vi "Register with Manager.vi"(8 "error in (no error)":errorcluster, 11 "CIFCorePlugin in":refnum<class "CIFCorePlugin.lvclass">) -> (0 "error out":errorcluster, 3 "CIFCorePlugin out":refnum<class "CIFCorePlugin.lvclass">)   [LabVIEW 2021, in "CIFCorePlugin.lvclass"]
uses:
  CIFCorePlugin.lvclass
  CIFPluginManager/CIFPluginManager/gRPC/CIF_Manager_client/RPC Messages/cif_manager_RegisterData.ctl
  CIFPluginManager/CIFPluginManager/gRPC/CIF_Manager_client/RPC Messages/cif_common_ShortVersion.ctl
  CIFCorePlugin.lvclass/CIFCorePlugin.ctl
  Common/Typedef/Errors.ctl
  <vilib>/gRPC/LabVIEW gRPC Library/Shared/grpcId.ctl
  <vilib>/CIF Foundation/CIF Utilities/Errors/Append Error Location.vi
  CIFPluginManager/CIFPluginManager/gRPC/CIF_Manager_Client_Wrapper/CIFManagerClientWrapper.lvlib
  CIFUtilities/CIFConfigurationFile/CIF Configuration File.lvlib
  CIFPluginManager/CIFPluginManager/gRPC/CIF_Manager_client/CIF_Manager_client.lvlib
  Common/CIFCoreCommon.lvlib
  <vilib>/gRPC/LabVIEW gRPC Library/grpc-lvsupport-release.lvlib
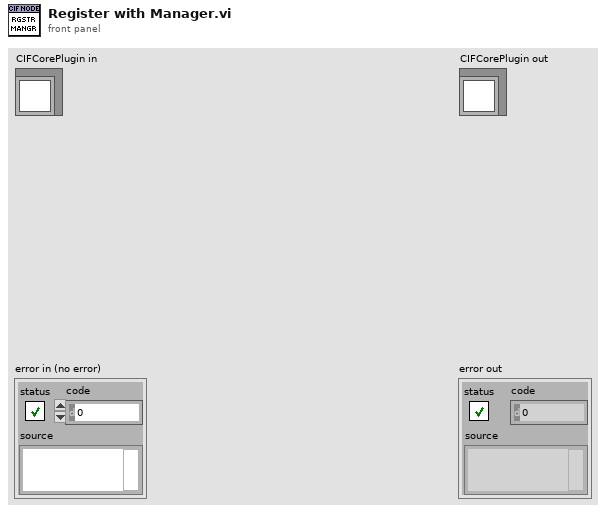
[diagram p1: front panel]
types:
  T1 = typedef "CIF_Manager_client.lvlib/cif_manager_RegisterData.ctl" = cluster{"plugin_name":string, "grpc_port":i32, "plugin_version":T2}
  T2 = typedef "CIF_Manager_client.lvlib/cif_common_ShortVersion.ctl" = cluster{"major":u32, "minor":u32, "fix":u32}
  T3 = typedef "grpc-lvsupport-release.lvlib/grpcId.ctl" = u64
  T4 = typedef "CIFCoreCommon.lvlib/Errors.ctl" = enum16{"Invalid Clock ID", "Long Sleep", "gRPC Server Not Found", "Config Parse", "Timestamp Wrap", "Delayed Execution", "Duplicate Channel", "Missing Channel", "Incorrect Type", "Flatten Error", "Unflatten Data", "Unique Name", "Plugin Not Found", "Plugin Type Not Found", "Plugin Version Not Found", "Manager Not Found", "Numerical Issue", "Time Jump", "Clock ID Match", "Channel Length", "Plugin Connection", "gRPC Server Connection", "PPL Name Match", "Build", "Config Log Parse", "Plugin Load", "UI Subpanel Load", "Python Name", "Invalid Name", "Unable to Change Ch Buffer"}
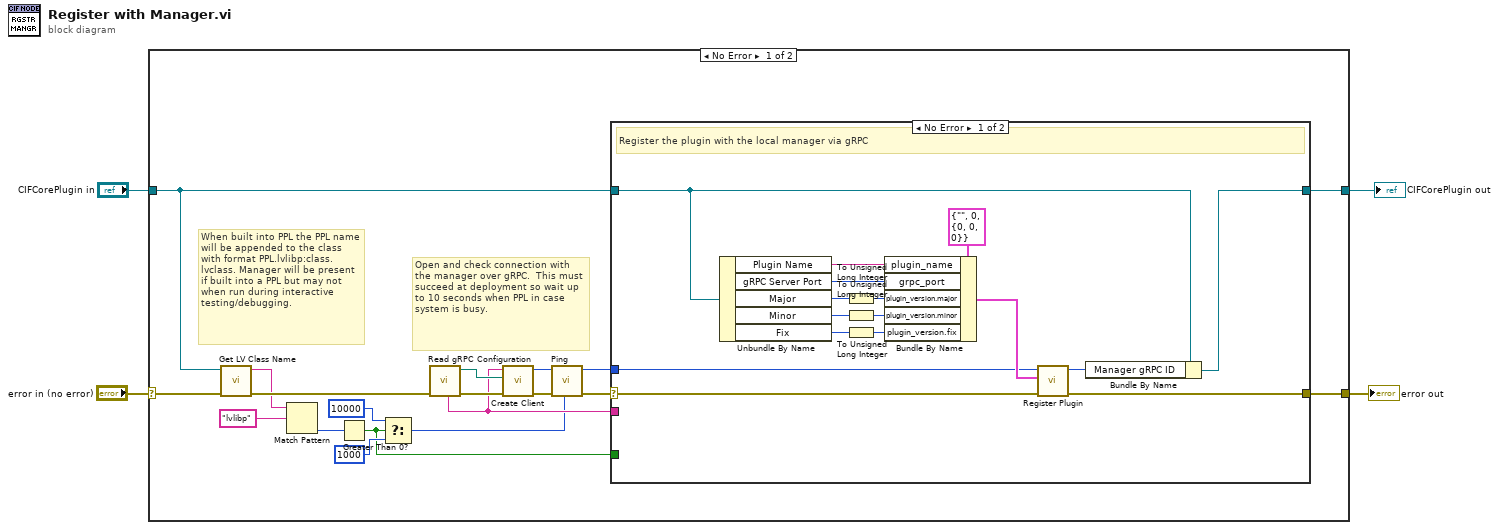
[diagram p0: block diagram]
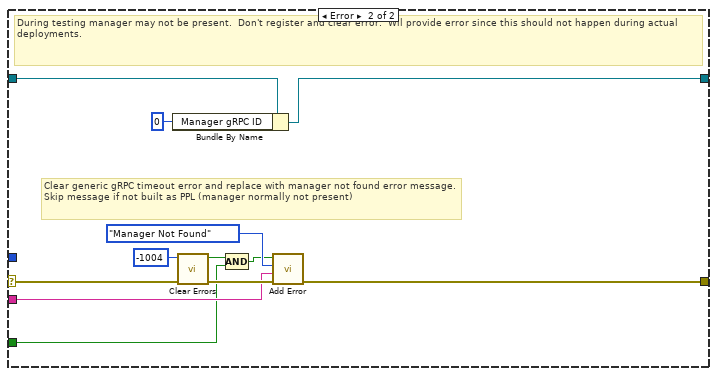
[diagram p2: hidden frame]
diagram:
  n1 = case shown="No Error" "error in (no error)" {
    selector: "error in (no error)" -> [w20 w53]
    tunnel: [w23 w53] -> w3
    tunnel: [w22 w52] -> w1
    tunnel: "CIFCorePlugin in" -> [w21 w52]
    frame No Error {
      # "Open and check connection with the manager over gRPC.  This must succeed at deployment so wait up to 10 seconds when PPL in case system is busy."
      # "When built into PPL the PPL name will be appended to the class with format PPL.lvlibp:class.lvclass. Manager will be present if built into a PPL but may not when run during interactive testing/debugging."
      n2 = call <vilib>:"Get LV Class Name.vi"("error in (no error)"=w20, "object"=w21) -> ("error out"=w19:errorcluster, "class name"=w18:string)  [unwired: 8 in]
      n3 = Match Pattern(string=w18, regular expression="lvlibp") -> (offset past match=w16:i32)  [unwired: 1 in, 3 out]
      n4 = Greater Than 0?(x=w16) -> (x > 0?=w5:bool)
      n5 = Select(t=10000 ("timeout (ms)"), s=w5, f=1000 ("timeout (ms)")) -> (s? t:f=w7:i32)
      n6 = call "Read gRPC Configuration.vi"("error in"=w19) -> ("error out"=w15:errorcluster, "Server Certificate File (.crt)"=w14:path, "Local Manager Address"=w9:string)  [unwired: 5 in, 3 out]
      n7 = call "Create Client.vi"("error in"=w15, "Server Certificate File (.crt)"=w14, "address"=w9) -> ("error out"=w13:errorcluster, "gRPC ID Out"=w12:T3)  [unwired: 7 in]
      n8 = call "Ping.vi"("timeout (ms)"=w7, "error in"=w13, "gRPC ID in"=w12) -> ("error out"=w11:errorcluster, "gRPC ID out"=w10:T3)  [unwired: 7 in]
      n9 = case shown="No Error" w11 {
        selector: w11 -> [w31 w48]
        tunnel: w10 -> [w32 _]
        tunnel: w21 -> [w30 w51]
        tunnel: [w27 w50] -> w22
        tunnel: [w28 w45] -> w23
        tunnel: w9 -> [_ w44]
        tunnel: w5 -> [_ w41]
        frame No Error {
          # "Register the plugin with the local manager via gRPC"
          n10 = Unbundle By Name(w30) -> ("Plugin Name"=w38:string, "gRPC Server Port"=w37:i32, "Major"=w36:i32, "Minor"=w34:i32, "Fix"=w35:i32)
          n11 = To Unsigned Long Integer(number=w36) -> (unsigned 32bit integer=w26:u32)
          n12 = To Unsigned Long Integer(number=w34) -> (unsigned 32bit integer=w25:u32)
          n13 = To Unsigned Long Integer(number=w35) -> (unsigned 32bit integer=w24:u32)
          n14 = Bundle By Name(cluster=T1 {"plugin_name"="", "grpc_port"=0, "plugin_version"={"major"=0, "minor"=0, "fix"=0}} ("Register"), "plugin_name"=w38, "grpc_port"=w37, "plugin_version.major"=w26, "plugin_version.minor"=w25, "plugin_version.fix"=w24) -> (w33:T1)
          n15 = call "Register Plugin.vi"("error in"=w31, "Register"=w33, "gRPC ID in"=w32) -> ("error out"=w28:errorcluster, "gRPC ID out"=w29:T3)  [unwired: 7 in]
          n16 = Bundle By Name(cluster=w30, "Manager gRPC ID"=w29) -> (w27:refnum<class "CIFCorePlugin.lvclass">)
        }
        frame Error {
          # "Clear generic gRPC timeout error and replace with manager not found error message.  Skip message if not built as PPL (manager normally not present)"
          # "During testing manager may not be present.  Don't register and clear error.  Wil provide error since this should not happen during actual deployments."
          n17 = Bundle By Name(cluster=w51, "Manager gRPC ID"=T3 0) -> (w50:refnum<class "CIFCorePlugin.lvclass">)
          n18 = call <vilib>:"Clear Errors.vi"("error in (no error)"=w48, "specific error code to clear (0: all)"=-1004) -> ("error out"=w46:errorcluster, "specific error cleared?"=w42:bool)  [unwired: 4 in]
          n19 = Compound Arithmetic op=AND(w42, w41) -> (w40:bool)
          n20 = call "Add Error.vi"("error in (no error)"=w46, "String to Append"=w44, "Error"=Errors."Manager Not Found", "Insert Error"=w40) -> ("error out"=w45:errorcluster)  [unwired: 7 in]
        }
      }
    }
    frame Error {
    }
  }
  "error out" <- w3
  "CIFCorePlugin out" <- w1
